vi "Pause P40.vi"(8 "error in (no error)":errorcluster, 11 "SSI P40 Settings In":T1={"VISA resource name"="", "Simulated?"=TRUE}) -> (0 "error out":errorcluster, 1 "Connection Error":bool, 3 "SSI P40 Settings Out":T1={"VISA resource name"="", "Simulated?"=TRUE})   [LabVIEW 2021, in "SSI P40 Pump.lvlib"]
uses:
  SSI P40 Pump.lvlib
  SSI P40 Settings Cluster.ctl
  SSI PR or LD Pump.lvlib
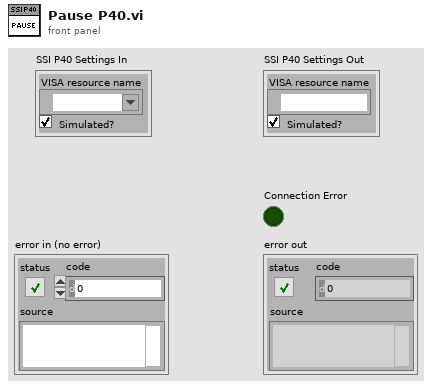
[diagram p1: front panel]
types:
  T1 = typedef "SSI P40 Pump.lvlib/SSI P40 Settings Cluster.ctl" = cluster{"VISA resource name":refnum<visa-resource-name>, "Simulated?":bool}
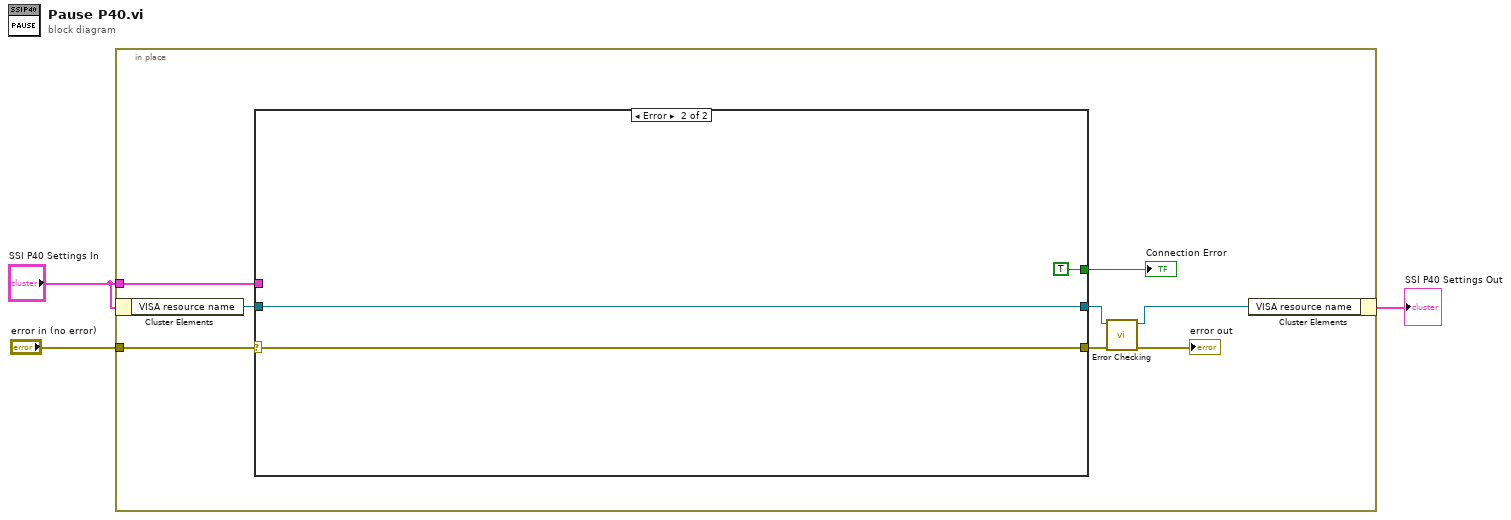
[diagram p0: block diagram]
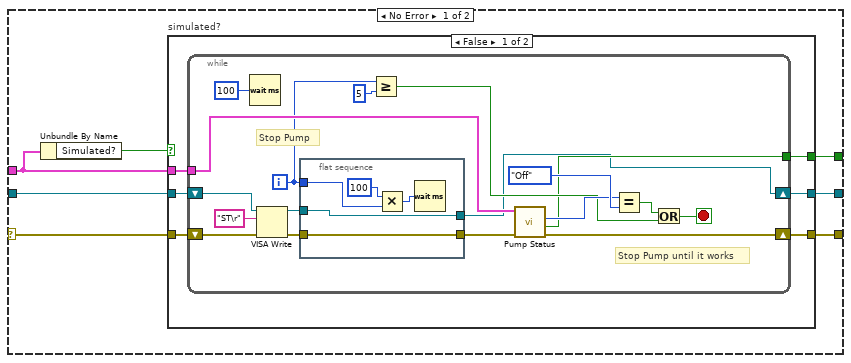
[diagram p2: hidden frame]
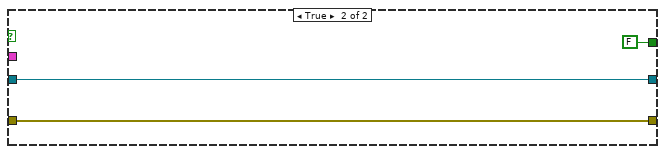
[diagram p3: hidden frame]
diagram:
  n1 = in-place {
    in-place-border: "SSI P40 Settings In" -> [w8]
    in-place-border: "error in (no error)" -> [w7]
    n2 = in-place-cluster #1("SSI P40 Settings In") -> ("VISA resource name"=w5:refnum<visa-resource-name>)
    n3 = case shown="Error" w7 {
      selector: w7 -> [w18 w53]
      tunnel: w8 -> [w15 _]
      tunnel: [w17 w51] -> w11
      tunnel: [w16 w53] -> w10
      tunnel: [w13 TRUE ("Connection Error")] -> w6
      tunnel: w5 -> [w12 w51]
      frame No Error {
        n4 = Unbundle By Name(w15) -> ("Simulated?"=w14:bool)
        n5 = case "simulated?" shown="False" w14 {
          tunnel: [w22 w50] -> w17
          tunnel: w12 -> [w24 w50]
          tunnel: w18 -> [w23 w49]
          tunnel: [w21 w49] -> w16
          tunnel: w15 -> [w20 _]
          tunnel: [w19 FALSE ("Connection Error")] -> w13
          frame False {
            n6 = while {
              shift-right: [w30] -> w22
              shift-left: w24 -> [w42]
              shift-right: [w37] -> w21
              shift-left: w23 -> [w41]
              tunnel: w20 -> [w36]
              tunnel: [w31] -> w19
              i -> [w26]
              stop <- w25 stop-if-true
              # "Stop Pump until it works"
              # "Stop Pump"
              n7 = Wait (ms)(milliseconds to wait=u32 100) -> ()  [unwired: 1 out]
              n8 = VISA Write(VISA resource name=w42, write buffer="ST\r" ("string"), error in (no error)=w41) -> (VISA resource name out=w29:refnum<visa-resource-name>, error out=w27:errorcluster)  [unwired: 1 out]
              n9 = flat-sequence {
                tunnel: [w47] -> w30
                tunnel: w29 -> [w47]
                tunnel: [w46] -> w28
                tunnel: w27 -> [w46]
                tunnel: w26 -> [w43]
                frame #0 {
                  n10 = Multiply(x=u32 100 ("milliseconds to wait"), y=w43) -> (x*y=w45:u32)
                  n11 = Wait (ms)(milliseconds to wait=w45) -> ()  [unwired: 1 out]
                }
              }
              n12 = Greater Or Equal?(x=w26, y=5) -> (x >= y?=w33:bool)
              n13 = call "Pump Status.vi"("error in (no error)"=w28, "SSI PR Settings"=w36) -> ("error out"=w37:errorcluster, "Connection Error"=w31:bool, "Pump On?"=w35:enum16{"Off", "On", "Not Initialized"})  [unwired: 4 in, 3 out]
              n14 = Equal?(x=w35, y=enum16{"Off", "On", "Not Initialized"}."Off") -> (x = y?=w32:bool)
              n15 = Or(x=w32, y=w33) -> (x .or. y?=w25:bool)
            }
          }
          frame True {
          }
        }
      }
      frame Error {
      }
    }
    "Connection Error" <- w6
    n16 = call "Error Checking.vi"("error in (no error)"=w10, "VISA resource name"=w11) -> ("error out"=→"error out":errorcluster, "VISA resource name"=w4:refnum<visa-resource-name>)  [unwired: 7 in, 1 out]
    n17 = in-place-cluster #1("VISA resource name"=w4) -> (→"SSI P40 Settings Out":T1)
  }
